vi "Merge Bilevel PWC Clusters.vi"(3 "error in (no error)":errorcluster, 4 "Max Gap Length":i32, 5 "Bilevel PWC Waveform":i32[](array[numeric])) -> (0 "error out":errorcluster, 2 "Merged Bilevel PWC Waveform":i32[](array[numeric]))   [LabVIEW 2012]
panel:
  out "Waveform Graph":i32[][](graph)
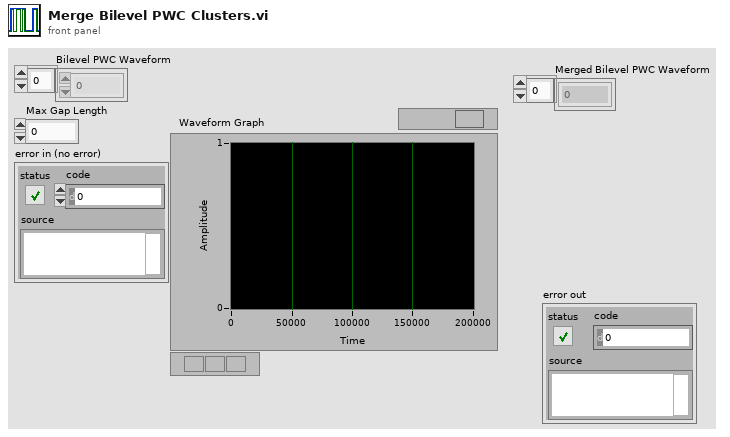
[diagram p1: front panel]
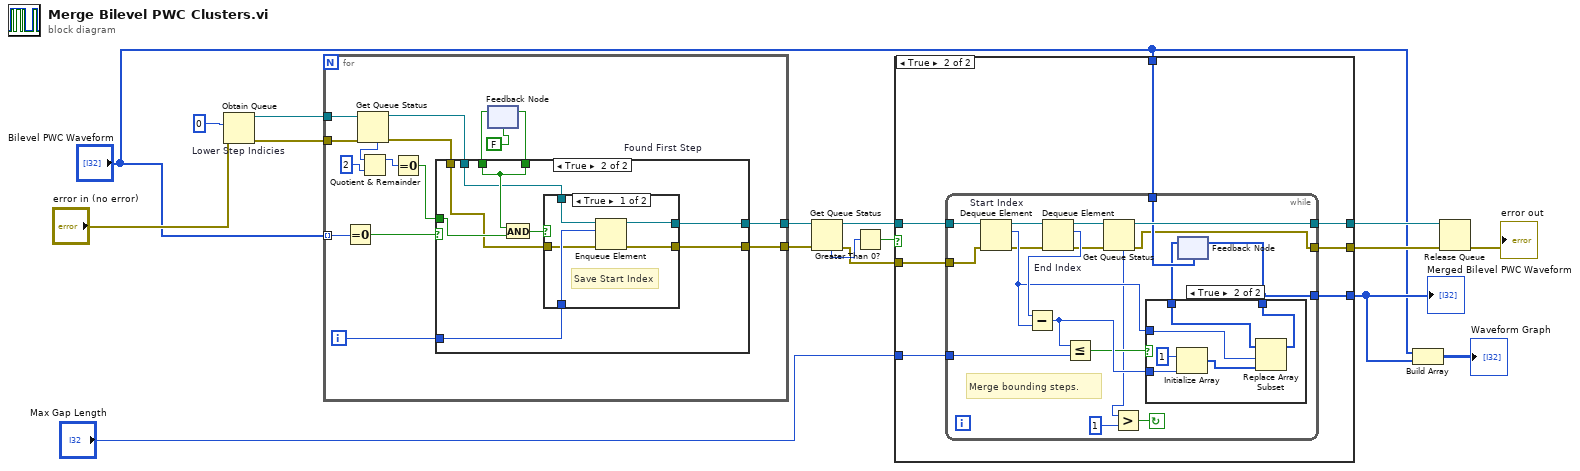
[diagram p0: block diagram]
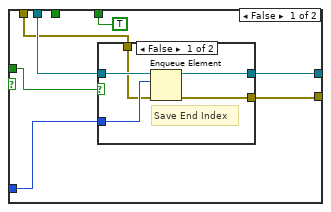
[diagram p4: hidden frame]
diagram:
  n1 = Obtain Queue "Lower Step Indicies"(element data type=0, error in (no error)="error in (no error)") -> (queue out=w17:refnum<queue>, error out=w9:errorcluster)  [unwired: 3 in, 1 out]
  n2 = for {
    tunnel: "Bilevel PWC Waveform" -> [w30] mode=indexing
    tunnel: w17 -> [w26]
    tunnel: [w31] -> w13
    tunnel: w9 -> [w20]
    tunnel: [w18] -> w8
    i -> [w29]
    n3 = Equal To 0?(x=w30) -> (x = 0?=w27:bool)
    n4 = Get Queue Status(queue=w26, error in (no error)=w20) -> (queue out=w25:refnum<queue>, error out=w19:errorcluster, # elements in queue=w21:i32)  [unwired: 1 in, 5 out]
    n5 = Quotient & Remainder(x=w21, y=2) -> (x-y*floor(x/y)=w23:i32)  [unwired: 1 out]
    n6 = Equal To 0?(x=w23) -> (x = 0?=w22:bool)
    n7 = feedback #1 "Found First Step"(FALSE) -> (w28:bool)
    n8 = case shown="True" w27 {
      tunnel: w28 -> [_ w53]
      tunnel: [TRUE w53] -> w32
      tunnel: [w37 w55] -> w31
      tunnel: w29 -> [w36 w54]
      tunnel: w25 -> [w38 w51]
      tunnel: w22 -> [w39 w50]
      tunnel: w19 -> [w35 w49]
      tunnel: [w34 w48] -> w18
      frame False {
        n9 = case shown="False" w39 {
          tunnel: w38 -> [w45 w47]
          tunnel: [w44 w47] -> w37
          tunnel: w36 -> [w43 _]
          tunnel: w35 -> [w42 w46]
          tunnel: [w41 w46] -> w34
          frame False {
            # "Save End Index"
            n10 = Enqueue Element(queue=w45, element=w43, error in (no error)=w42) -> (queue out=w44:refnum<queue>, error out=w41:errorcluster)  [unwired: 1 in, 1 out]
          }
          frame True {
          }
        }
      }
      frame True {
        n11 = And(x=w53, y=w50) -> (x .and. y?=w52:bool)
        n12 = case shown="True" w52 {
          tunnel: w51 -> [w60 w62]
          tunnel: [w59 w62] -> w55
          tunnel: w54 -> [w58 _]
          tunnel: w49 -> [w57 w61]
          tunnel: [w56 w61] -> w48
          frame True {
            # "Save Start Index"
            n13 = Enqueue Element(queue=w60, element=w58, error in (no error)=w57) -> (queue out=w59:refnum<queue>, error out=w56:errorcluster)  [unwired: 1 in, 1 out]
          }
          frame False {
          }
        }
      }
    }
    n14 = feedback-in #1(w32) -> ()
  }
  n15 = Get Queue Status(queue=w13, error in (no error)=w8) -> (queue out=w11:refnum<queue>, error out=w7:errorcluster, # elements in queue=w12:i32)  [unwired: 1 in, 5 out]
  n16 = Greater Than 0?(x=w12) -> (x > 0?=w14:bool)
  n17 = case shown="True" w14 {
    tunnel: [w65 w72] -> w15
    tunnel: w11 -> [w65 w68]
    tunnel: "Bilevel PWC Waveform" -> [w64 w71]
    tunnel: [w64 w70] -> w3
    tunnel: "Max Gap Length" -> [_ w69]
    tunnel: w7 -> [w63 w67]
    tunnel: [w63 w66] -> w6
    frame False {
    }
    frame True {
      n18 = while {
        tunnel: w68 -> [w90]
        tunnel: [w87] -> w72
        tunnel: w71 -> [w84]
        tunnel: [w79] -> w70
        tunnel: w69 -> [w82]
        tunnel: w67 -> [w76]
        tunnel: [w73] -> w66
        stop <- w91 continue-if-true
        # "Merge bounding steps."
        n19 = Dequeue Element "Start Index"(queue=w90, error in (no error)=w76) -> (queue out=w89:refnum<queue>, element=w85:i32, error out=w75:errorcluster)  [unwired: 1 in, 1 out]
        n20 = Dequeue Element "End Index"(queue=w89, error in (no error)=w75) -> (queue out=w88:refnum<queue>, element=w86:i32, error out=w74:errorcluster)  [unwired: 1 in, 1 out]
        n21 = Subtract(x=w86, y=w85) -> (x-y=w83:i32)
        n22 = Less Or Equal?(x=w83, y=w82) -> (x <= y?=w81:bool)
        n23 = Get Queue Status(queue=w88, error in (no error)=w74) -> (queue out=w87:refnum<queue>, error out=w73:errorcluster, # elements in queue=w78:i32)  [unwired: 1 in, 5 out]
        n24 = Greater?(x=w78, y=1) -> (0:w91:bool)
        n25 = feedback #2(w84) -> (w80:i32[])
        n26 = case shown="True" w81 {
          tunnel: w83 -> [_ w96]
          tunnel: w85 -> [_ w95]
          tunnel: [w92 w94] -> w79
          tunnel: w80 -> [w92 w93]
          frame False {
          }
          frame True {
            n27 = Initialize Array(1, w96) -> (w97:i32[])
            n28 = Replace Array Subset(array=w93, new element=w97, index=w95) -> (w94:i32[])
          }
        }
        n29 = feedback-in #2(w79) -> ()
      }
    }
  }
  "Merged Bilevel PWC Waveform" <- w3
  n30 = Build Array("Bilevel PWC Waveform", w3) -> (→"Waveform Graph":i32[][])
  n31 = Release Queue(queue=w15, error in (no error)=w6) -> (error out=→"error out":errorcluster)  [unwired: 1 in, 2 out]
